vi "TDMS Logger.vi"() -> ()   [LabVIEW 2018]
uses:
  <vilib>/Utility/error.llb/Error Cluster From Error Code.vi
  <vilib>/ErrorRing/Error Ring.xnode
panel:
  out "Power Spectrum":waveform(dbl)[](graph)
  out "Time Data":waveform(dbl)[](graph)
  in  "UUT Serial Numbers":string[](array[string])
  in  "Test Operator":string
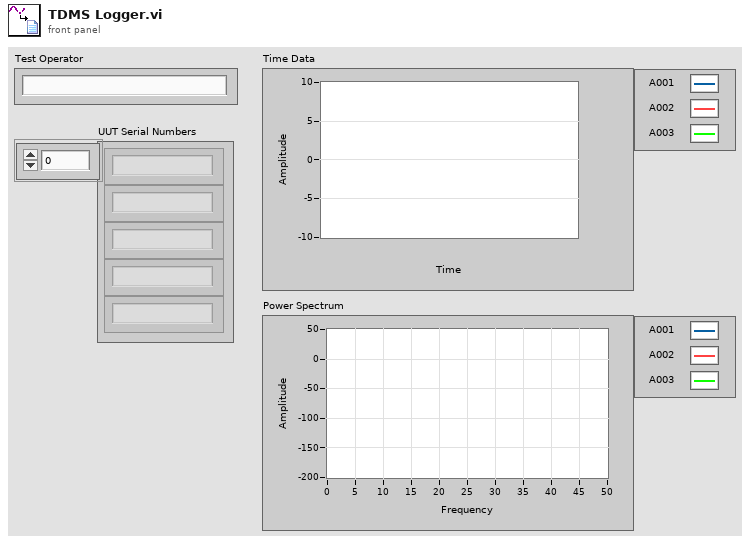
[diagram p1: front panel]
types:
  T1 = enum16{"open", "open or create", "create or replace", "create", "open (read-only)"}
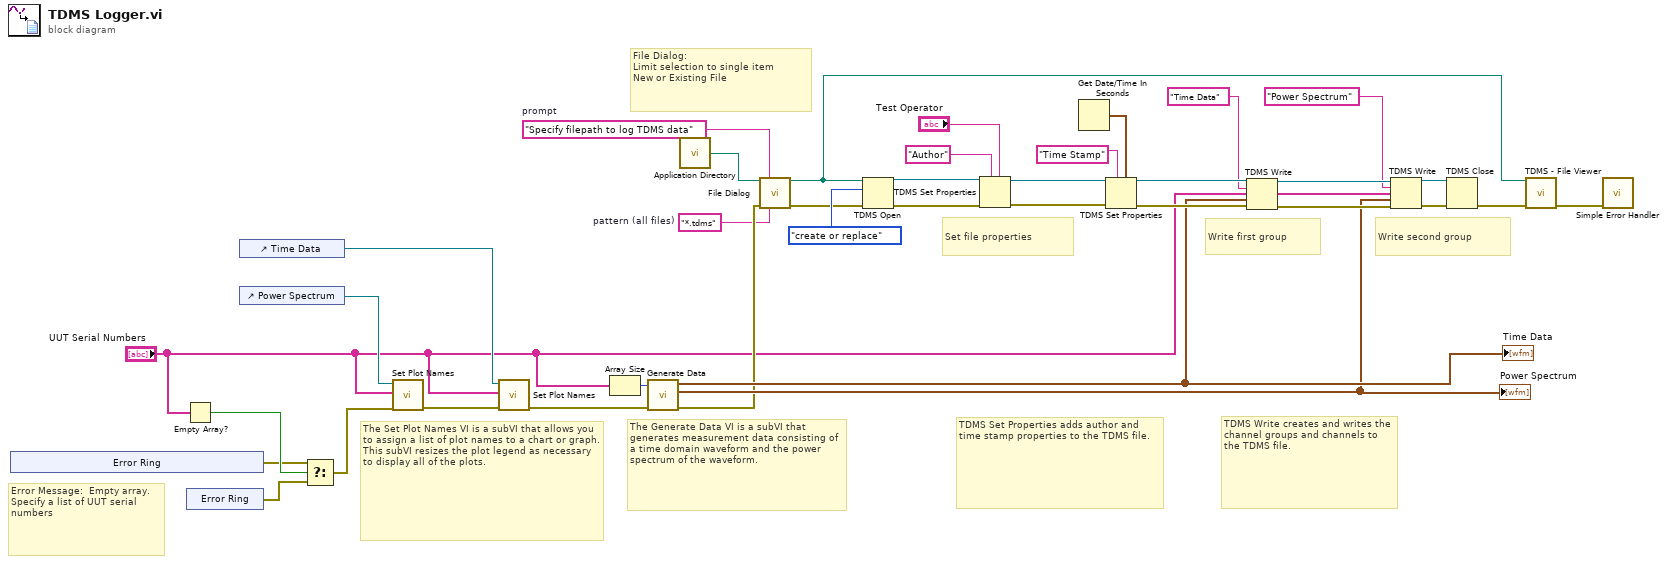
[diagram p0: block diagram]
diagram:
  w9 = "*.tdms"  # pattern (all files)
  w13 = "Specify filepath to log TDMS data"  # prompt
  # "Error Message:  Empty array. Specify a list of UUT serial numbers"
  # "File Dialog:\nLimit selection to single item\nNew or Existing File"
  # "Write second group"
  # "Write first group"
  # "Set file properties"
  # "TDMS Set Properties adds author and time stamp properties to the TDMS file."
  # "TDMS Write creates and writes the channel groups and channels to the TDMS file."
  # "The Generate Data VI is a subVI that generates measurement data consisting of a time domain waveform and the power spectrum of the waveform."
  # "The Set Plot Names VI is a subVI that allows you to assign a list of plot names to a chart or graph.\nThis subVI resizes the plot legend as necessary to display all of the plots."
  n1 = xnode "Error Ring"() -> ("error out"=w2:errorcluster)
  n2 = Empty Array?(array="UUT Serial Numbers") -> (empty?=w6:bool)
  n3 = xnode "Error Ring"() -> ("error out"=w3:errorcluster)
  n4 = control-ref of="Time Data"() -> (w15:refnum<vi>)
  n5 = control-ref of="Power Spectrum"() -> (w16:refnum<vi>)
  n6 = Select(t=w2, s=w6, f=w3) -> (s? t:f=w4:errorcluster)
  n7 = call "Set Plot Names.vi"("error in"=w4, "Plot Names"="UUT Serial Numbers", "Graph Reference"=w16) -> ("error out"=w38:errorcluster)  [unwired: 8 in]
  n8 = call "Set Plot Names.vi"("error in"=w38, "Plot Names"="UUT Serial Numbers", "Graph Reference"=w15) -> ("error out"=w5:errorcluster)  [unwired: 8 in]
  n9 = Array Size(array="UUT Serial Numbers") -> (size(s)=w37:i32)
  n10 = call "Generate Data.vi"("error in"=w5, "Number of Channels"=w37) -> ("error out"=w11:errorcluster, "Power Spectrum"=w17:waveform(dbl)[], "Time Data"=w18:waveform(dbl)[])  [unwired: 7 in]
  "Time Data" <- w18
  "Power Spectrum" <- w17
  n11 = call <vilib>:"Application Directory.vi"() -> ("Application Directory"=w12:path)
  n12 = call "File Dialog"("start path"=w12, "prompt"=w13, "error in"=w11, "pattern (all files)"=w9) -> ("selected path"=w14:path, "error out"=w10:errorcluster)  [unwired: 8 in, 2 out]
  n13 = TDMS Open(8:w10, 10:T1."create or replace" ("operation (0:open)"), 11:w14) -> (0:w30:errorcluster, 3:w35:refnum<k34>)  [unwired: 4 in]
  n14 = TDMS Set Properties(5:"Test Operator", 7:"Author", 8:w30, 11:w35) -> (0:w34:errorcluster, 3:w33:refnum<k34>)  [unwired: 2 in, 2 out]
  n15 = Get Date/Time In Seconds() -> (seconds since 1Jan1904=w31:timestamp)
  n16 = TDMS Set Properties(5:w31, 7:"Time Stamp" ("Title"), 8:w34, 11:w33) -> (0:w28:errorcluster, 3:w29:refnum<k34>)  [unwired: 2 in, 2 out]
  n17 = TDMS Write(0:w29, 5:"Time Data" ("group name in (Untitled)"), 7:"UUT Serial Numbers", 9:w18, 11:w28) -> (4:w27:refnum<k34>, 8:w24:string[], 15:w26:errorcluster)  [unwired: 1 in, 1 out]
  n18 = TDMS Write(0:w27, 5:"Power Spectrum" ("group name in (Untitled)"), 7:w24, 9:w17, 11:w26) -> (4:w23:refnum<k34>, 15:w22:errorcluster)  [unwired: 1 in, 2 out]
  n19 = TDMS Close(8:w22, 11:w23) -> (0:w21:errorcluster)  [unwired: 1 out]
  n20 = call <vilib>:"TDMS - File Viewer.vi"("error in (no error)"=w21, "file path"=w14) -> ("error out"=w20:errorcluster)  [unwired: 4 in, 1 out]
  n21 = call <vilib>:"Simple Error Handler.vi"("error in (no error)"=w20) -> ()  [unwired: 4 in, 5 out]
